vi "Send Query.vi"(6 "Big Data?":bool, 8 "error in":errorcluster, 10 "Query":string, 11 "3300 in":refnum<class "3300.lvclass">) -> (0 "error out":errorcluster, 2 "Read Data":string, 3 "3300 out":refnum<class "3300.lvclass">)   [LabVIEW 2019, in "3300.lvlib" / "3300.lvclass"]
uses:
  Library/3300.lvclass
  Library/3300.lvclass/3300.ctl
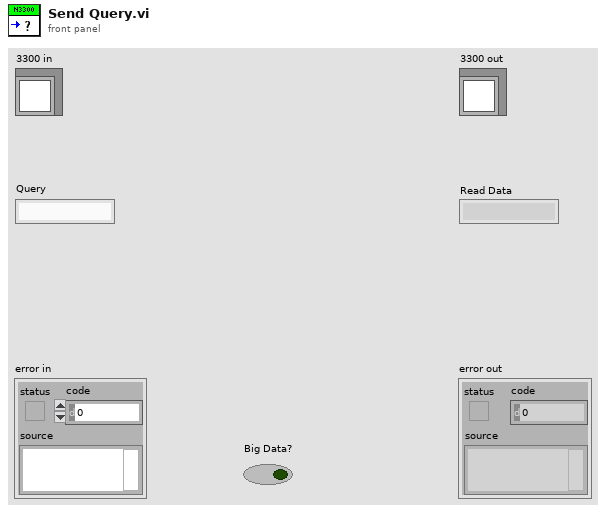
[diagram p1: front panel]
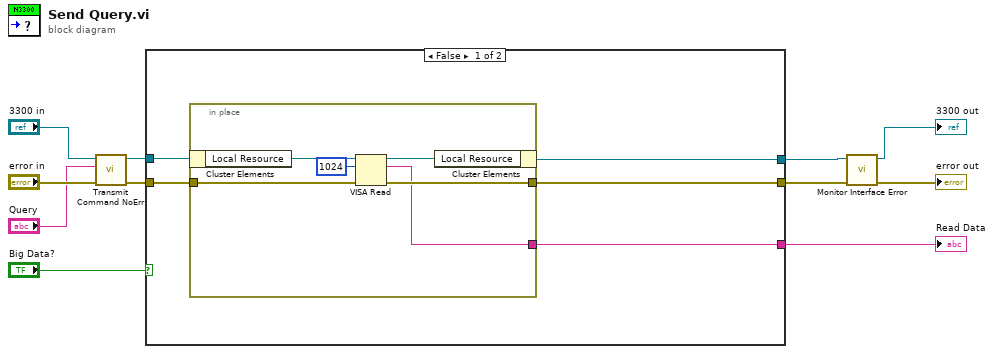
[diagram p0: block diagram]
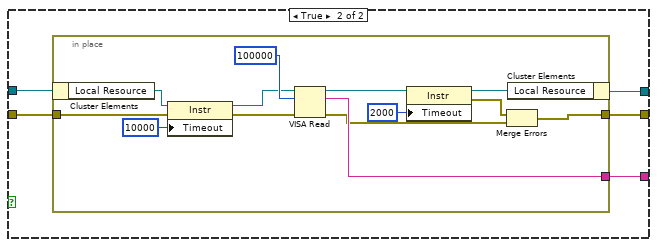
[diagram p2: hidden frame]
diagram:
  n1 = call "Transmit Command NoErr.vi"("error in"="error in", "Command"="Query", "3300 in"="3300 in") -> ("error out"=w9:errorcluster, "3300 out"=w8:refnum<class "3300.lvclass">)  [unwired: 7 in]
  n2 = case shown="False" "Big Data?" {
    tunnel: [w16 w27] -> w4
    tunnel: [w15 w26] -> w3
    tunnel: [w14 w25] -> w11
    tunnel: w9 -> [w13 w24]
    tunnel: w8 -> [w12 w23]
    frame False {
      n3 = in-place {
        in-place-border: w13 -> [w20]
        in-place-border: [w19] -> w15
        in-place-border: [w18] -> w14
        n4 = in-place-cluster #1(w12) -> ("Local Resource"=w22:refnum<visa-resource-name>)
        n5 = VISA Read(VISA resource name=w22, byte count=u32 1024, error in (no error)=w20) -> (VISA resource name out=w21:refnum<visa-resource-name>, read buffer=w18:string, error out=w19:errorcluster)  [unwired: 1 out]
        n6 = in-place-cluster #1("Local Resource"=w21) -> (w16:refnum<class "3300.lvclass">)
      }
    }
    frame True {
      n7 = in-place {
        in-place-border: w24 -> [w36]
        in-place-border: [w29] -> w26
        in-place-border: [w40] -> w25
        n8 = in-place-cluster #2(w23) -> ("Local Resource"=w37:refnum<visa-resource-name>)
        n9 = property class="Instr"(reference=w37, error in=w36, "Timeout"=u32 10000 ("General Settings:Timeout Value")) -> (reference out=w35:refnum<visa-resource-name>, error out=w34:errorcluster)
        n10 = VISA Read(VISA resource name=w35, byte count=u32 100000, error in (no error)=w34) -> (VISA resource name out=w32:refnum<visa-resource-name>, read buffer=w40:string, error out=w28:errorcluster)  [unwired: 1 out]
        n11 = property class="Instr"(reference=w32, "Timeout"=u32 2000 ("General Settings:Timeout Value")) -> (reference out=w31:refnum<visa-resource-name>, error out=w30:errorcluster)  [unwired: 1 in]
        n12 = Merge Errors(w30, w28) -> (w29:errorcluster)
        n13 = in-place-cluster #2("Local Resource"=w31) -> (w27:refnum<class "3300.lvclass">)
      }
    }
  }
  "Read Data" <- w11
  n14 = call "Monitor Interface Error.vi"("error in"=w3, "3300 in"=w4) -> ("error out"=→"error out":errorcluster, "3300 out"=→"3300 out":refnum<class "3300.lvclass">)  [unwired: 8 in]
